vi "Check XML File against XSD Schema.vi"(8 "error in (no error)":errorcluster, 10 "XML Configuration File Path":path=path "E:/Ballard - Arinc-429 CD/Example Database/Ballard/XML_000.XML", 11 "XML Schema File Path":path=path "E:/Ballard - Arinc-429 CD/Source/System Explorer/SubVIs/Parse XML Ballard/BTI.XSD") -> (0 "error IO":errorcluster)   [LabVIEW 2016, in "Ballard Arinc-429 System Explorer.lvlib"]
uses:
  Ballard Arinc-429 System Explorer.lvlib
  C:/Users/Vincent/Desktop/Ballard-Arinc-429-Custom-Device Inline Async/Source/System Explorer/SubVIs/Parse XML Ballard/Ballard_BTI_XML_Deserializer.dll
  Ballard_BTI_XML_Deserializer.dll
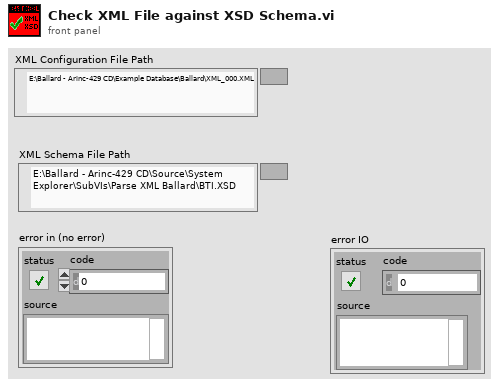
[diagram p1: front panel]
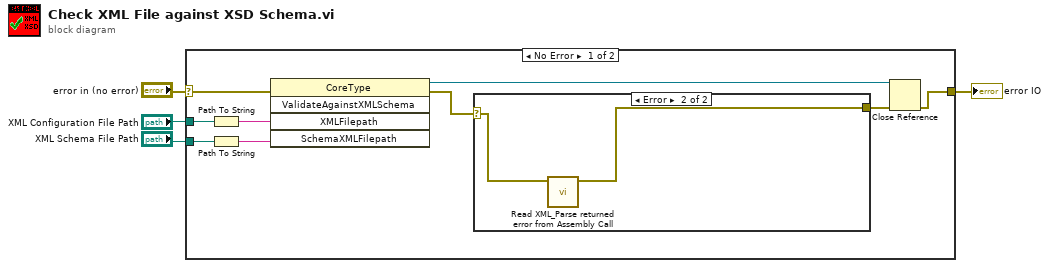
[diagram p0: block diagram]
diagram:
  n1 = case shown="No Error" "error in (no error)" {
    selector: "error in (no error)" -> [w7 w17]
    tunnel: "XML Configuration File Path" -> [w13 _]
    tunnel: "XML Schema File Path" -> [w12 _]
    tunnel: [w9 w17] -> w1
    frame No Error {
      n2 = Path To String(path=w13) -> (string=w6:string)
      n3 = Path To String(path=w12) -> (string=w11:string)
      n4 = invoke class="CoreType" method="ValidateAgainstXMLSchema"(error in=w7, "XMLFilepath"=w6, "SchemaXMLFilepath"=w11) -> (reference out=w8:refnum<k24>, error out=w5:errorcluster)  [unwired: 2 in, 3 out]
      n5 = case shown="Error" w5 {
        selector: w5 -> [w14 w16]
        tunnel: [w14 w15] -> w10
        frame No Error {
        }
        frame Error {
          n6 = call "Read XML_Parse returned error from Assembly Call.vi"("error in (no error)"=w16) -> ("error out"=w15:errorcluster)  [unwired: 10 in]
        }
      }
      n7 = Close Reference(reference=w8, error in (no error)=w10) -> (error out=w9:errorcluster)
    }
    frame Error {
    }
  }
  "error IO" <- w1
